vi "angular feed forward.vi"(8 "sensor units":dbl=8192.0, 10 "force gain":dbl=1.0, 11 "position":dbl) -> (3 "power":dbl=1.0 format="%#_6f")   [LabVIEW 2020]
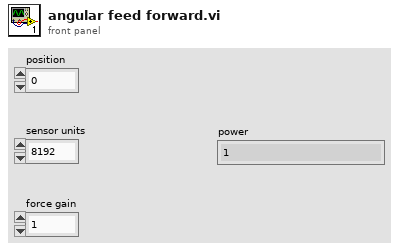
[diagram p1: front panel]
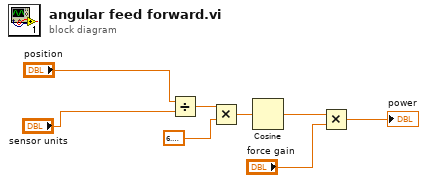
[diagram p0: block diagram]
diagram:
  n1 = Divide(x="position", y="sensor units") -> (x/y=w6:dbl)
  n2 = Multiply(x=w6, y=6.283185307179586) -> (x*y=w4:dbl)
  n3 = Cosine(x=w4) -> (cos(x)=w3:dbl)
  n4 = Multiply(x=w3, y="force gain") -> (x*y=→"power":dbl)
